vi "modify control module.vi"(6 "output range":cluster{"output high":dbl, "output low":dbl}={"output high"=100.0, "output low"=-100.0}, 8 "error in":errorcluster, 9 "gains":T1, 10 "name":string, 11 "user module configuration in":refnum<class "fixed channel tag bus module configuration.lvclass">) -> (0 "error out":errorcluster, 3 "user module configuration out":refnum<class "fixed channel tag bus module configuration.lvclass">)   [LabVIEW 2013]
uses:
  <vilib>/NI/Tag Bus Module Framework/root configuration/TBM configuration.lvclass
  fixed channel tag bus module configuration.lvclass
  gains.ctl
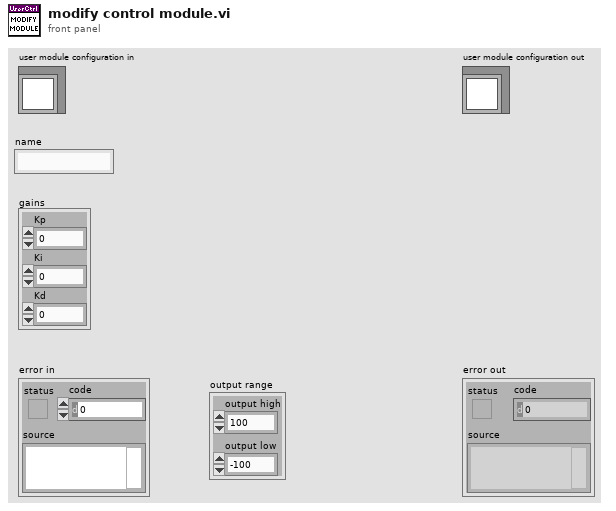
[diagram p1: front panel]
types:
  T1 = typedef "gains.ctl" = cluster{"Kp":dbl, "Ki":dbl, "Kd":dbl}
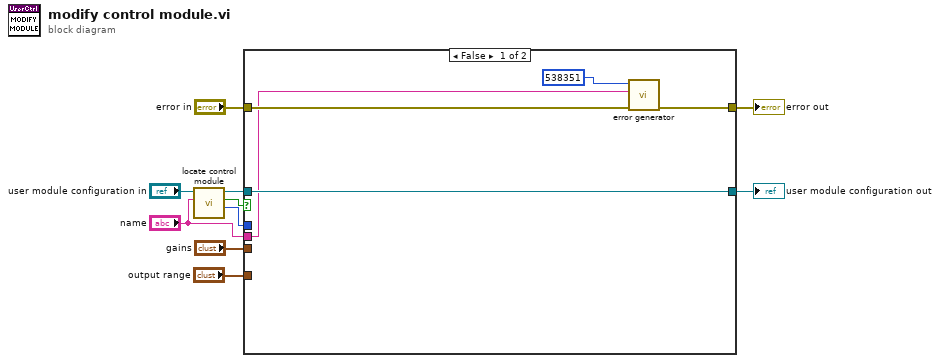
[diagram p0: block diagram]
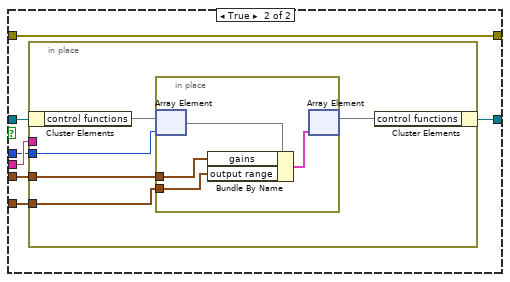
[diagram p2: hidden frame]
diagram:
  n1 = call "locate control module.vi"("name"="name", "user module configuration in"="user module configuration in") -> ("index"=w1:i32, "found"=w8:bool, "user module configuration out"=w9:refnum<class "fixed channel tag bus module configuration.lvclass">)  [unwired: 6 in, 1 out]
  n2 = case shown="False" w8 {
    tunnel: w9 -> [w12 w22]
    tunnel: "error in" -> [w15 w20]
    tunnel: [w13 w20] -> w6
    tunnel: [w12 w21] -> w5
    tunnel: "name" -> [w11 w19]
    tunnel: "output range" -> [_ w18]
    tunnel: "gains" -> [_ w17]
    tunnel: w1 -> [_ w16]
    frame False {
      n3 = call <vilib>:"error generator.vi"("error in"=w15, "append error message"=w11, "error code (0)"=538351) -> ("error out"=w13:errorcluster)  [unwired: 6 in]
    }
    frame True {
      n4 = in-place {
        in-place-border: w19 -> [_]
        in-place-border: w18 -> [w25]
        in-place-border: w17 -> [w24]
        in-place-border: w16 -> [w23]
        n5 = in-place-cluster #1(w22) -> ("control functions"=w27)
        n6 = in-place {
          in-place-border: w25 -> [w29]
          in-place-border: w24 -> [w28]
          n7 = in-place-array #2(w27, w23) -> (w31)
          n8 = Bundle By Name(cluster=w31, "gains"=w28, "output range"=w29) -> (w30:cluster{})
          n9 = in-place-array #2(w30) -> (w26)  [unwired: 1 out]
        }
        n10 = in-place-cluster #1("control functions"=w26) -> (w21:refnum<class "fixed channel tag bus module configuration.lvclass">)
      }
    }
  }
  "error out" <- w6
  "user module configuration out" <- w5
